vi "removeLastContinuation.vi"(11 "String in":string) -> (3 "String out":string)   [LabVIEW 2012]
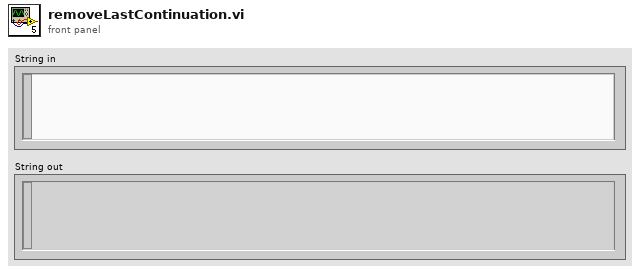
[diagram p1: front panel]
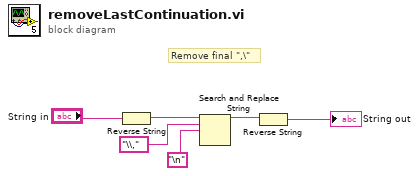
[diagram p0: block diagram]
diagram:
  # "Remove final \",\\\""
  n1 = Reverse String(1:"String in") -> (0:w5:string)
  n2 = Search and Replace String(input string=w5, search string="\\," ("search string/char (-)"), replace string="\n") -> (result string=w4:string)  [unwired: 5 in, 3 out]
  n3 = Reverse String(1:w4) -> (0:→"String out":string)
